vi "AlliGator Get Phasor Ratio Interpolated Color v2.vi"(4 "Color 2":T2, 6 "Color 1":T2, 7 "Color Fading?":bool, 8 "Error In":errorcluster, 9 "Phasor Ratio/Average Lifetime Display Range":cluster{"Min":dbl, "Max":dbl}={"Min"=0.0, "Max"=1.0}, 10 "-d_0":sgl, 11 "Phasor Ratio Data":T1) -> (0 "Error Out":errorcluster, 1 "Transparent?":bool, 3 "Overlay Color":T2)   [LabVIEW 2021, in "AlliGator Phasor Ratio.lvlib"]
doc: "Computes phasor ratio equivalent color using the two references' colors."
uses:
  AlliGator Phasor Ratio.lvlib
  AlliGator Phasor Ratio Data.ctl
panel:
  # "see the AlliGator License on the block diagram (Ctrl+E or Window:Show Block Diagram)"
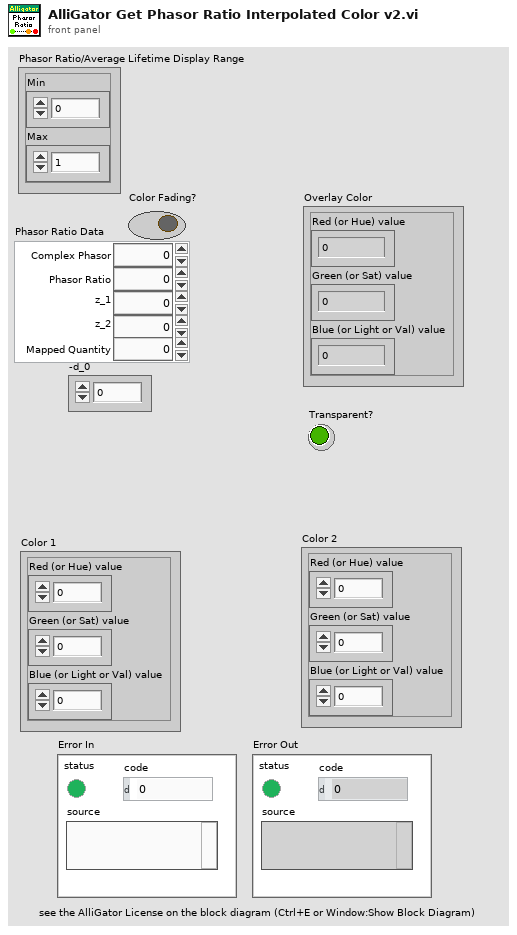
[diagram p1: front panel]
types:
  T1 = typedef "AlliGator Phasor Ratio.lvlib/AlliGator Phasor Ratio Data.ctl" = cluster{"Complex Phasor":csg, "Phasor Ratio":sgl, "z_1":csg, "z_2":csg, "Mapped Quantity":sgl}
  T2 = cluster{"Red (or Hue) value":u8, "Green (or Sat) value":u8, "Blue (or Light or Val) value":u8}
  T3 = cluster{"Red (or Hue) value":dbl, "Green (or Sat) value":dbl, "Blue (or Light or Val) value":dbl}
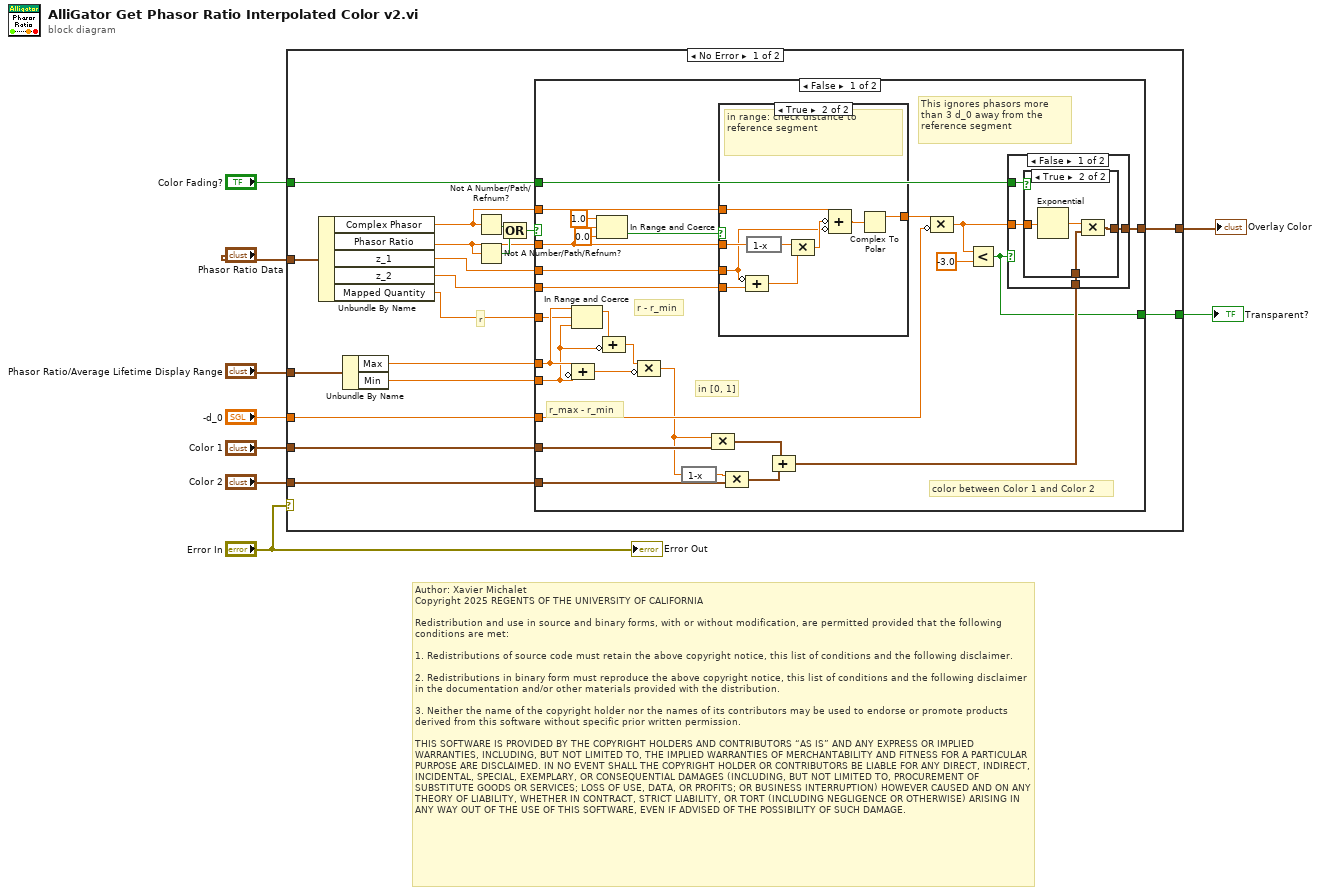
[diagram p0: block diagram]
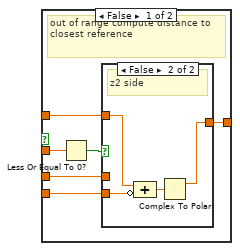
[diagram p4: hidden frame]
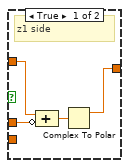
[diagram p5: hidden frame]
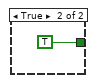
[diagram p6: hidden frame]
diagram:
  # "Author: Xavier Michalet\nCopyright 2025 REGENTS OF THE UNIVERSITY OF CALIFORNIA\n\nRedistribution and use in source and binary forms, with or without modification, are permitted provided that the following conditions are met:\n\n1. Redistributions of source code must retain the above copyright notice, this list of conditions and the following disclaimer.\n\n2. Redistributions in binary form must reproduce the above copyright notice, this list of conditions and the following disclaimer in the documentation and/or other materials provided with the distribution.\n\n3. Neither the name of the copyright holder nor the names of its contributors may be used to endorse or promote products derived from this software without specific prior written permission.\n\nTHIS SOFTWARE IS PROVIDED BY THE COPYRIGHT HOLDERS AND CONTRIBUTORS “AS IS” AND ANY EXPRESS OR IMPLIED WARRANTIES, INCLUDING, BUT NOT LIMITED TO, THE IMPLIED WARRANTIES OF MERCHANTABILITY AND FITNESS FOR A PARTICULAR PURPOSE ARE DISCLAIMED. IN NO EVENT SHALL THE COPYRIGHT HOLDER OR CONTRIBUTORS BE LIABLE FOR ANY DIRECT, INDIRECT, INCIDENTAL, SPECIAL, EXEMPLARY, OR CONSEQUENTIAL DAMAGES (INCLUDING, BUT NOT LIMITED TO, PROCUREMENT OF SUBSTITUTE GOODS OR SERVICES; LOSS OF USE, DATA, OR PROFITS; OR BUSINESS INTERRUPTION) HOWEVER CAUSED AND ON ANY THEORY OF LIABILITY, WHETHER IN CONTRACT, STRICT LIABILITY, OR TORT (INCLUDING NEGLIGENCE OR OTHERWISE) ARISING IN ANY WAY OUT OF THE USE OF THIS SOFTWARE, EVEN IF ADVISED OF THE POSSIBILITY OF SUCH DAMAGE."
  n1 = case shown="No Error" "Error In" {
    tunnel: "Color 2" -> [w27 _]
    tunnel: "Color 1" -> [w26 _]
    tunnel: "-d_0" -> [w25 _]
    tunnel: [w24 _] -> w6
    tunnel: [w23 _] -> w5
    tunnel: "Color Fading?" -> [w22 _]
    tunnel: "Phasor Ratio Data" -> [w18 _]
    tunnel: "Phasor Ratio/Average Lifetime Display Range" -> [w13 _]
    frame No Error {
      # "r"
      n2 = Unbundle By Name(w18) -> ("Complex Phasor"=w17:csg, "Phasor Ratio"=w16:sgl, "z_1"=w15:csg, "z_2"=w14:csg, "Mapped Quantity"=w10:sgl)
      n3 = Unbundle By Name(w13) -> ("Max"=w12:dbl, "Min"=w11:dbl)
      n4 = Not A Number/Path/Refnum?(number/path/refnum=w17) -> (NaN/Path/Refnum?=w21:bool)
      n5 = Not A Number/Path/Refnum?(number/path/refnum=w16) -> (NaN/Path/Refnum?=w20:bool)
      n6 = Compound Arithmetic op=OR(w21, w20) -> (w19:bool)
      n7 = case shown="False" w19 {
        tunnel: w15 -> [w54 _]
        tunnel: w14 -> [w53 _]
        tunnel: w27 -> [w51 _]
        tunnel: w26 -> [w50 _]
        tunnel: w25 -> [w46 _]
        tunnel: [w44 _] -> w24
        tunnel: [w43 TRUE] -> w23
        tunnel: w22 -> [w41 _]
        tunnel: w17 -> [w40 _]
        tunnel: w16 -> [w31 _]
        tunnel: w12 -> [w36 _]
        tunnel: w11 -> [w35 _]
        tunnel: w10 -> [w34 _]
        frame False {
          # "r - r_min"
          # "r_max - r_min"
          # "color between Color 1 and Color 2"
          # "in [0, 1]"
          # "This ignores phasors more than 3 d_0 away from the reference segment"
          n8 = In Range and Coerce(upper limit=w36, x=w34, lower limit=w35) -> (coerced(x)=w39:dbl)  [unwired: 1 out]
          n9 = Compound Arithmetic op=ADD(w36, invert w35) -> (w38:dbl)
          n10 = In Range and Coerce(upper limit=sgl 1.0, x=w31, lower limit=sgl 0.0) -> (In Range?=w28:bool)  [unwired: 1 out]
          n11 = Compound Arithmetic op=ADD(w39, invert w35) -> (w37:dbl)
          n12 = Compound Arithmetic op=MULTIPLY(w37, invert w38) -> (w33:dbl)
          n13 = expression code="1-x"(w33) -> (w32:dbl)
          n14 = Compound Arithmetic op=MULTIPLY(w33, w50) -> (w49:T3)
          n15 = case shown="True" w28 {
            tunnel: w40 -> [w67 w86]
            tunnel: w54 -> [w66 w80]
            tunnel: w31 -> [w69 w85]
            tunnel: [w65 w82] -> w52
            tunnel: w53 -> [w64 w81]
            frame False {
              # "out of range compute distance to closest reference"
              n16 = Less Or Equal To 0?(x=w69) -> (x <= 0?=w68:bool)
              n17 = case shown="False" w68 {
                tunnel: w67 -> [w73 w77]
                tunnel: w66 -> [w72 _]
                tunnel: [w70 w75] -> w65
                tunnel: w64 -> [_ w74]
                frame True {
                  # "z1 side"
                  n18 = Compound Arithmetic op=ADD(w73, invert w72) -> (w71:csg)
                  n19 = Complex To Polar(r * e^(i*theta)=w71) -> (r=w70:sgl)  [unwired: 1 out]
                }
                frame False {
                  # "z2 side"
                  n20 = Compound Arithmetic op=ADD(w77, invert w74) -> (w76:csg)
                  n21 = Complex To Polar(r * e^(i*theta)=w76) -> (r=w75:sgl)  [unwired: 1 out]
                }
              }
            }
            frame True {
              # "in range: check distance to reference segment"
              n22 = Compound Arithmetic op=ADD(invert w80, w81) -> (w79:csg)
              n23 = expression code="1-x"(w85) -> (w78:sgl)
              n24 = Compound Arithmetic op=MULTIPLY(w78, w79) -> (w84:csg)
              n25 = Compound Arithmetic op=ADD(w86, invert w84, invert w80) -> (w83:csg)
              n26 = Complex To Polar(r * e^(i*theta)=w83) -> (r=w82:sgl)  [unwired: 1 out]
            }
          }
          n27 = Compound Arithmetic op=MULTIPLY(w32, w51) -> (w48:T3)
          n28 = Compound Arithmetic op=ADD(w49, w48) -> (w47:T3)
          n29 = Compound Arithmetic op=MULTIPLY(w52, invert w46) -> (w45:sgl)
          n30 = Less?(x=w45, y=sgl -3.0) -> (x < y?=w43:bool)
          n31 = case shown="False" w43 {
            tunnel: w47 -> [w58 _]
            tunnel: w45 -> [w57 _]
            tunnel: [w56 _] -> w44
            tunnel: w41 -> [w55 _]
            frame False {
              n32 = case shown="True" w55 {
                tunnel: w58 -> [w59 w63]
                tunnel: w57 -> [_ w61]
                tunnel: [w59 w60] -> w56
                frame False {
                }
                frame True {
                  n33 = Exponential(1:w61) -> (0:w62:sgl)
                  n34 = Compound Arithmetic op=MULTIPLY(w62, w63) -> (w60:T3)
                }
              }
            }
            frame True {
            }
          }
        }
        frame True {
        }
      }
    }
    frame Error {
    }
  }
  "Overlay Color" <- w6
  "Transparent?" <- w5
  "Error Out" <- "Error In"
